vi "chords.vi"(10 "Notenames":string[](array[string]), 11 "Notes in Scale":bool[](array[boolean])) -> (0 "MIDI-values":string[][](array[string]), 1 "Chord Frequencies":dbl[][][](array[numeric]), 3 "Chords":string[][](array[string]))   [LabVIEW 2019]
uses:
  <vilib>/Utility/file.llb/Read Delimited Spreadsheet (string).vi
panel:
  out "all rows":string[][](array[string])
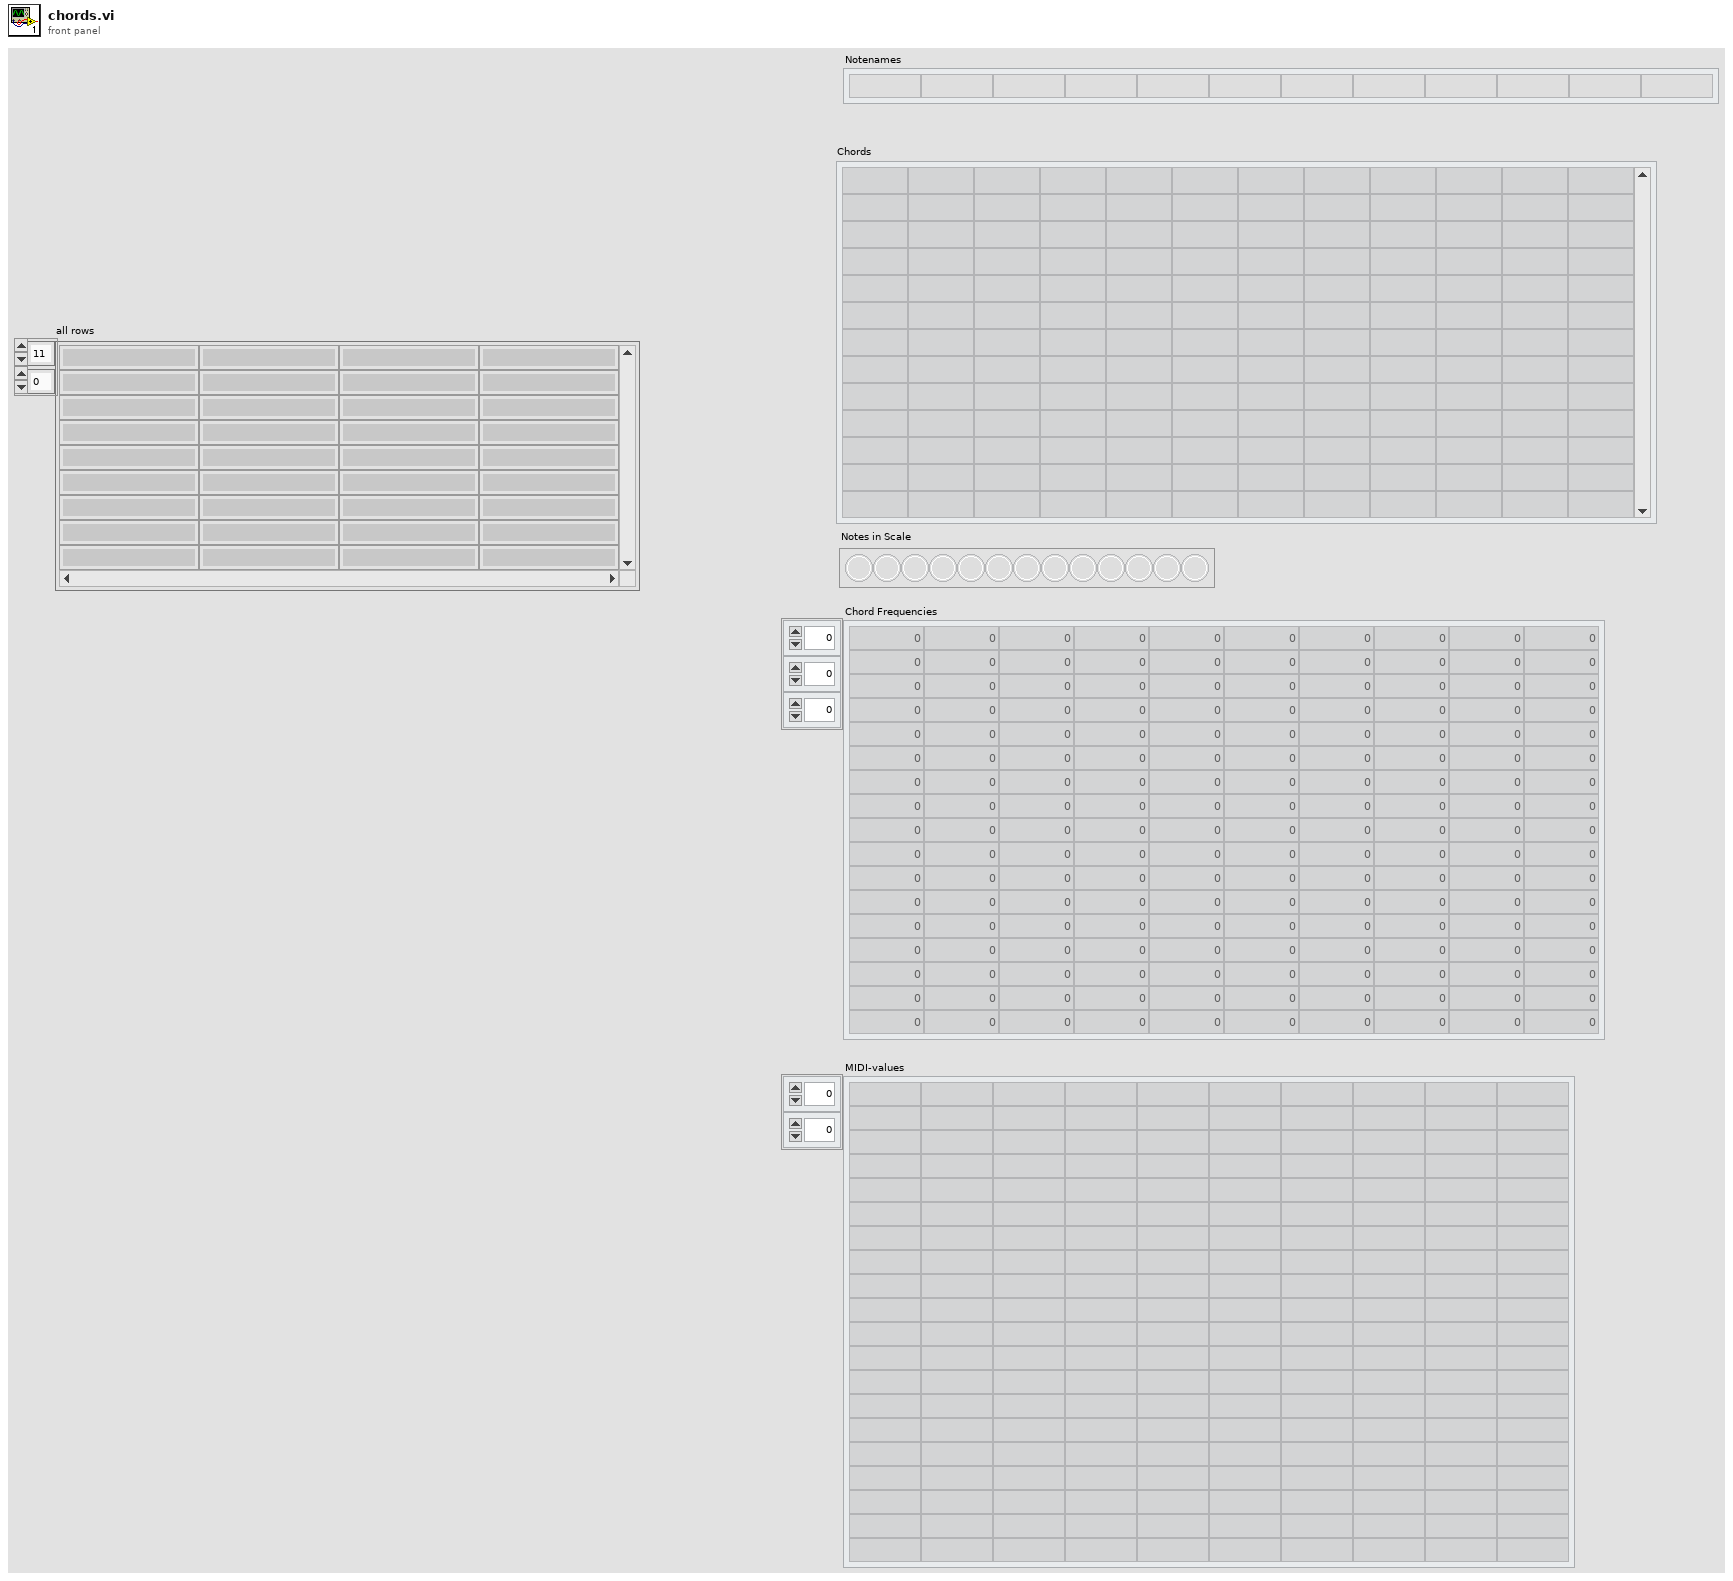
[diagram p1: front panel]
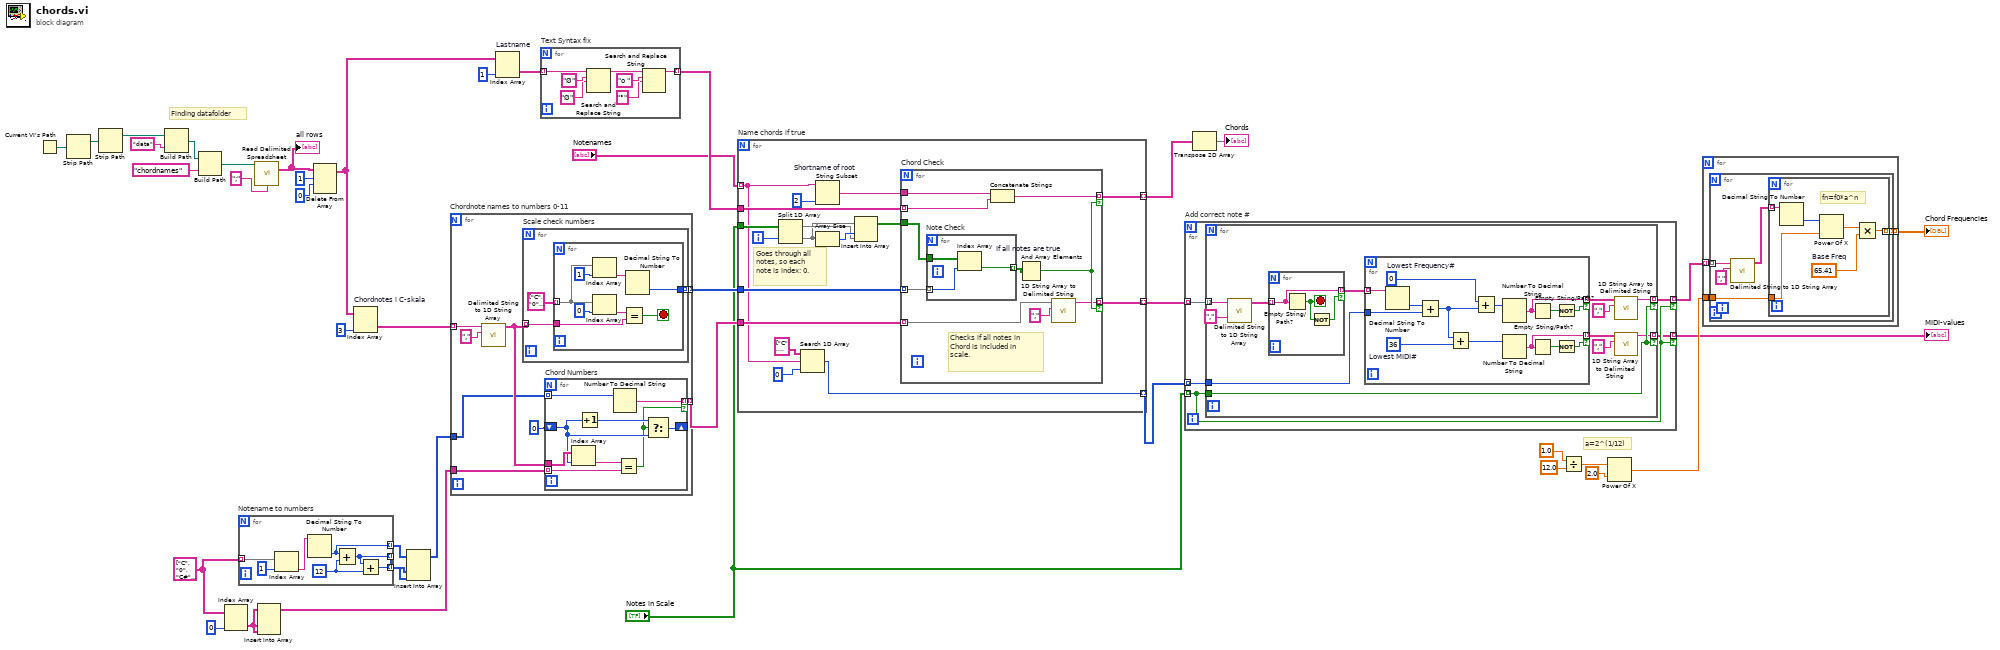
[diagram p0: block diagram]
diagram:
  w15 = string[][] [["C", "0"], ["C#", "1"], ["Db", "1"], ["D", "2"], ["D#", "3"], ["Eb", "3"], ["E", "4"], ["F", "5"], ["F#", "6"], ["Gb", "6"], ["G", "7"], ["G#", "8"], ["Ab", "8"], ["A", "9"], ["A#", "10"], ["Bb", "10"], ["B", "11"]]
  # "a=2^(1/12)"
  # "Finding datafolder"
  n1 = Current VI's Path() -> (path=w40:path)
  n2 = Strip Path ("Relative Path")(path=w40) -> (stripped path=w36:path)  [unwired: 1 out]
  n3 = Strip Path ("Relative Path")(path=w36) -> (stripped path=w35:path)  [unwired: 1 out]
  n4 = Build Path ("datafiles")(base path=w35, name or relative path="data") -> (appended path=w37:path)
  n5 = Build Path(base path=w37, name or relative path="chordnames") -> (appended path=w34:path)
  n6 = Index Array(array=w15, index (col)=0 ("index (row)")) -> (element=w19:string[])  [unwired: 1 in]
  n7 = for "Notename to numbers" {
    tunnel: w15 -> [w48] mode=indexing
    tunnel: [w44] -> w23 mode=indexing
    tunnel: [w43] -> w22 mode=indexing
    tunnel: [w42] -> w21 mode=indexing
    w45 = 12 ("y")
    n8 = Index Array(array=w48, index=1) -> (element=w46:string)
    n9 = Decimal String To Number(string=w46) -> (number=w44:i32)  [unwired: 2 in, 1 out]
    n10 = Add(x=w44, y=w45) -> (x+y=w43:i32)
    n11 = Add(x=w43, y=w45) -> (x+y=w42:i32)
  }
  n12 = call-poly <vilib>:"Read Delimited Spreadsheet.vi"("file path (dialog if empty)"=w34, "delimiter (\\t)"=";" ("delimiter (\\t)")) -> ("all rows"=w29:string[][])  [unwired: 8 in, 5 out]
  "all rows" <- w29
  n13 = Insert Into Array(array=w19, new element #1=w19, new element #2=w19) -> (w17:string[])  [unwired: 1 in]
  n14 = Delete From Array(array=w29, length=1, index (row)=0) -> (array with subset deleted=w28:string[][])  [unwired: 1 in, 1 out]
  n15 = Index Array "Chordnotes i C-skala"(array=w28, index (col)=3 ("index (row)")) -> (element=w20:string[])  [unwired: 1 in]
  n16 = Insert Into Array(array=w23, new element #1=w22, new element #2=w21) -> (w16:i32[])  [unwired: 1 in]
  n17 = for "Chordnote names to numbers 0-11" {
    tunnel: w20 -> [w56] mode=indexing
    tunnel: [w54] -> w27 mode=indexing
    tunnel: w17 -> [w51]
    tunnel: w16 -> [w50]
    tunnel: [w49] -> w14 mode=indexing
    n18 = call <vilib>:"Delimited String to 1D String Array.vi"("delimiter"=",", "delimited string"=w56) -> ("string array"=w52:string[])  [unwired: 9 in]
    n19 = for "Scale check numbers" {
      tunnel: w52 -> [w67] mode=indexing
      tunnel: [w66] -> w54 mode=indexing
      n20 = for {
        tunnel: string[][] [["C", "0"], ["C#", "1"], ["Db", "1"], ["D", "2"], ["D#", "3"], ["Eb", "3"], ["E", "4"], ["F", "5"], ["F#", "6"], ["Gb", "6"], ["G", "7"], ["G#", "8"], ["Ab", "8"], ["A", "9"], ["A#", "10"], ["Bb", "10"], ["B", "11"]] -> [w74] mode=indexing
        tunnel: w67 -> [w72]
        tunnel: [w69] -> w66
        stop <- w71 stop-if-true
        n21 = Index Array(array=w74, index=1) -> (element=w70:string)
        n22 = Index Array(array=w74, index=0) -> (element=w75:string)
        n23 = Equal?(x=w75, y=w72) -> (x = y?=w71:bool)
        n24 = Decimal String To Number(string=w70) -> (number=w69:i32)  [unwired: 2 in, 1 out]
      }
    }
    n25 = for "Chord Numbers" {
      tunnel: w52 -> [w63]
      shift-right: [w61] -> _
      shift-left: 0 -> [w62]
      tunnel: w51 -> [w60] mode=indexing
      tunnel: w50 -> [w58] mode=indexing
      tunnel: [w57] -> w49 mode=indexing if=w59
      n26 = Index Array(array=w63, index=w62) -> (element=w64:string)
      n27 = Increment(x=w62) -> (x+1=w65:i32)
      n28 = Number To Decimal String(number=w58) -> (decimal integer string=w57:string)  [unwired: 1 in]
      n29 = Equal?(x=w64, y=w60) -> (x = y?=w59:bool)
      n30 = Select(t=w65, s=w59, f=w62) -> (s? t:f=w61:i32)
    }
  }
  n31 = Index Array "Lastname"(array=w28, index (col)=1 ("index (row)")) -> (element=w26:string[])  [unwired: 1 in]
  n32 = for "Text Syntax fix" {
    tunnel: w26 -> [w83] mode=indexing
    tunnel: [w77] -> w25 mode=indexing
    n33 = Search and Replace String(input string=w83, search string="Ø", replace string="Ø" ("replace string (\"\")")) -> (result string=w80:string)  [unwired: 5 in, 3 out]
    n34 = Search and Replace String(input string=w80, search string="o ", replace string="°" ("replace string (\"\")")) -> (result string=w77:string)  [unwired: 5 in, 3 out]
  }
  n35 = for "Name chords if true" {
    tunnel: "Notes in Scale" -> [w98]
    tunnel: "Notenames" -> [w86] mode=indexing
    tunnel: w27 -> [w95]
    tunnel: w25 -> [w94]
    tunnel: [w84] -> w9 mode=indexing
    tunnel: w14 -> [w89]
    tunnel: [w90] -> w12 mode=indexing
    tunnel: [w85] -> w11 mode=indexing
    i -> [w91]
    # "Goes through all notes, so each note is index: 0."
    n36 = Split 1D Array(array=w98, index=w91) -> (first subarray=w99:bool[], second subarray=w97:bool[])
    n37 = Search 1D Array(1D array=string[] ["C", "C# / Db", "D", "D# / Eb", "E", "F", "F# / Gb", "G", "G# / Ab", "A", "A# / Bb", "B"] ("Notenames 2"), element=w86, start index (0)=0) -> (index of element=w85:i32)
    n38 = String Subset "Shortname of root"(string=w86, length (rest)=2 ("length (rest)")) -> (substring=w92:string)  [unwired: 1 in]
    n39 = Array Size(array=w97) -> (size(s)=w100:i32)
    n40 = Insert Into Array(array=w97, index=w100, new element=w99) -> (w96:bool[])
    n41 = for "Chord Check" {
      tunnel: w95 -> [w105] mode=indexing
      tunnel: w96 -> [w110]
      tunnel: w92 -> [w108]
      tunnel: w94 -> [w107] mode=indexing
      tunnel: [w106] -> w84 mode=indexing if=w104
      tunnel: w89 -> [w101] mode=indexing
      tunnel: [w102] -> w90 mode=indexing if=w104
      # "Checks if all notes in Chord is included in scale."
      n42 = for "Note Check" {
        tunnel: w105 -> [w113] mode=indexing
        tunnel: w110 -> [w112]
        tunnel: [w111] -> w109 mode=indexing
        n43 = Index Array(array=w112, index=w113) -> (element=w111:bool)
      }
      n44 = Concatenate Strings(w108, w107) -> (w106:string)
      n45 = And Array Elements "If all notes are true"(Boolean array=w109) -> (logical AND=w104:bool)
      n46 = call <vilib>:"1D String Array to Delimited String.vi"("delimiter"=",", "string array"=w101) -> ("delimited string"=w102:string)  [unwired: 9 in]
    }
  }
  n47 = for "Add correct note #" {
    tunnel: w12 -> [w118] mode=indexing
    tunnel: w11 -> [w117] mode=indexing
    tunnel: [w115] -> w8 mode=indexing if=w116
    tunnel: [w114] -> w1 mode=indexing if=w116
    tunnel: "Notes in Scale" -> [w116] mode=indexing
    n48 = for {
      tunnel: w118 -> [w129] mode=indexing
      tunnel: w117 -> [w127]
      tunnel: [w122] -> w115 mode=indexing if=w125
      tunnel: [w119] -> w114 mode=indexing if=w125
      tunnel: w116 -> [w125]
      n49 = call <vilib>:"Delimited String to 1D String Array.vi"("delimiter"=",", "delimited string"=w129) -> ("string array"=w128:string[])  [unwired: 9 in]
      n50 = for {
        tunnel: w128 -> [w147] mode=indexing
        tunnel: [w147] -> w126 mode=indexing if=w145
        stop <- w146 stop-if-true
        n51 = Empty String/Path?(string/path=w147) -> (empty?=w146:bool)
        n52 = Not(x=w146) -> (.not. x?=w145:bool)
      }
      n53 = for {
        tunnel: w127 -> [w143]
        tunnel: [w131] -> w121 mode=indexing if=w132
        tunnel: w126 -> [w139] mode=indexing
        tunnel: [w137] -> w124 mode=indexing if=w135
        w140 = 0  # Lowest Frequency#
        w142 = 36  # Lowest MIDI#
        n54 = Decimal String To Number(string=w139) -> (number=w144:i32)  [unwired: 2 in, 1 out]
        n55 = Add(x=w144, y=w143) -> (x+y=w141:i32)
        n56 = Add(x=w141, y=w142) -> (x+y=w134:i32)
        n57 = Add(x=w140, y=w141) -> (x+y=w138:i32)
        n58 = Number To Decimal String(number=w138) -> (decimal integer string=w137:string)  [unwired: 1 in]
        n59 = Number To Decimal String(number=w134) -> (decimal integer string=w131:string)  [unwired: 1 in]
        n60 = Empty String/Path?(string/path=w137) -> (empty?=w136:bool)
        n61 = Empty String/Path?(string/path=w131) -> (empty?=w133:bool)
        n62 = Not(x=w136) -> (.not. x?=w135:bool)
        n63 = Not(x=w133) -> (.not. x?=w132:bool)
      }
      n64 = call <vilib>:"1D String Array to Delimited String.vi"("delimiter"=",", "string array"=w124) -> ("delimited string"=w122:string)  [unwired: 9 in]
      n65 = call <vilib>:"1D String Array to Delimited String.vi"("delimiter"=",", "string array"=w121) -> ("delimited string"=w119:string)  [unwired: 9 in]
    }
  }
  "MIDI-values" <- w1
  n66 = Transpose 2D Array(2D array=w9) -> (transposed array=→"Chords":string[][])
  n67 = Divide(x=1.0, y=12.0) -> (x/y=w6:dbl)
  n68 = Power Of X(1:2.0 ("x"), 2:w6) -> (0:w3:dbl)
  n69 = for {
    tunnel: w8 -> [w150] mode=indexing
    tunnel: w3 -> [w149]
    tunnel: [w148] -> w2 mode=indexing
    n70 = for {
      tunnel: w150 -> [w155] mode=indexing
      tunnel: w149 -> [w152]
      tunnel: [w151] -> w148 mode=indexing
      n71 = call <vilib>:"Delimited String to 1D String Array.vi"("delimiter"=",", "delimited string"=w155) -> ("string array"=w153:string[])  [unwired: 9 in]
      n72 = for {
        tunnel: w153 -> [w161] mode=indexing
        tunnel: w152 -> [w159]
        tunnel: [w158] -> w151 mode=indexing
        w156 = 65.41  # Base Freq
        # "fn=f0*a^n"
        n73 = Decimal String To Number(string=w161) -> (number=w157:i32)  [unwired: 2 in, 1 out]
        n74 = Power Of X(1:w159, 2:w157) -> (0:w160:dbl)
        n75 = Multiply(x=w160, y=w156) -> (x*y=w158:dbl)
      }
    }
  }
  "Chord Frequencies" <- w2
